vi "ADCS.UnlockECUSecurity.vi"(6 "Diagnostic Protocol":T2, 8 "error in (no error)":errorcluster, 10 "Security":T1={"Source DLL Path"=path "", "Security Level"=1, "Target DLL Path"=path ""}, 11 "diag ref in":T3) -> (0 "error out":errorcluster, 1 "success?":bool, 3 "diag ref out":T3)   [LabVIEW 2015, in "Diagnostics Addon Engine.lvlib"]
uses:
  Diagnostics Addon Engine.lvlib
  <vilib>/Automotive Diagnostic Command Set/Diagnostic Transport.llb/Diag Reference.ctl
  <vilib>/Automotive Diagnostic Command Set/Diagnostic Transport.llb/Transport Protocol Selector.ctl
  <vilib>/Automotive Diagnostic Command Set/Diagnostic Transport.llb/Diag CAN Frame Log.ctl
  Shared/Types/Protocol.ctl
  Shared/Types/Security.ctl
  GMLAN/_SubVIs/SecurityAccess_sendKey.vi
  GMLAN/_SubVIs/SecurityAccess_requestSeed.vi
  <vilib>/Automotive Diagnostic Command Set/Diagnostic Transport.llb/Apply Success Failure Error.vi
  <vilib>/Automotive Diagnostic Command Set/Diagnostic Transport.llb/Diagnostic Service.vi
  GMLAN/GMLAN.lvlib
  <vilib>/addons/Automotive Diagnostic Command Set/NI_Automotive Diagnostic Command Set.lvlib
  Shared/Diagnostics Addon Shared.lvlib
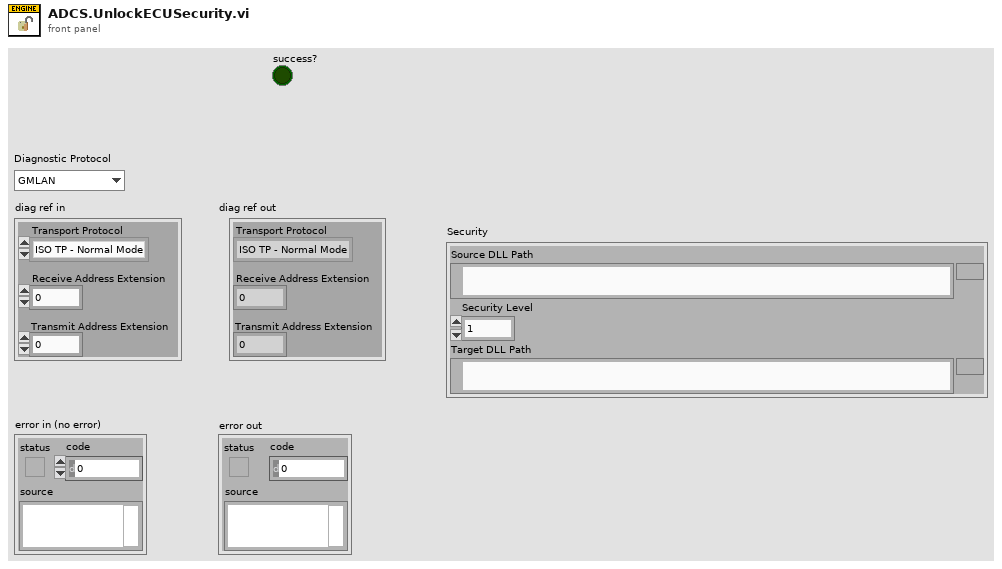
[diagram p1: front panel]
types:
  T1 = typedef "Diagnostics Addon Shared.lvlib/Security.ctl" = cluster{"Source DLL Path":path, "Security Level":u8, "Target DLL Path":path}
  T2 = typedef "Diagnostics Addon Shared.lvlib/Protocol.ctl" = enum16{"GMLAN", "KWP-2000", "UDS", "User-Defined"}
  T3 = typedef "NI_Automotive Diagnostic Command Set.lvlib/Diag Reference.ctl" = cluster{"Diag CAN Handle":u32, "Transport Protocol":T4, "Receive Address Extension":u8, "Transmit Address Extension":u8, "Receive CAN Id":u32, "Transmit CAN Id":u32, "Diag CAN Queue":refnum<queue>, "Log Frames ?":bool, "My TP Address":u8, "Other TP Address":u8, "T1":u16, "T2":u16, "T3":u16, "T4":u16, "Tx SN":u8, "Block Size":u8, "Rx SN":u8, "VW TP Initialized?":bool, "Tx block no":u8, "baud rate":u32, "Interface":string, "Channel Diag CAN Handle":u32, "UDP Connection ID":refnum<k16>, "TCP Connection ID":refnum<k5>, "Target IP Addr":u32, "Source Address":u16, "Target Address":u16, "Send Header NACK?":bool, "DLL Handle":u32, "NAD":u8, "Time Stamp read first":dbl, "Time Stamp read last":dbl, "Time Stamp write first":dbl, "Time Stamp write last":dbl, "Time Stamp write":dbl, "Time Stamp read":dbl}
  T4 = typedef "NI_Automotive Diagnostic Command Set.lvlib/Transport Protocol Selector.ctl" = enum16{"ISO TP - Normal Mode", "ISO TP - Mixed Mode", "VW TP 2.0", "Diagnostics on IP", "ISO TP LIN"}
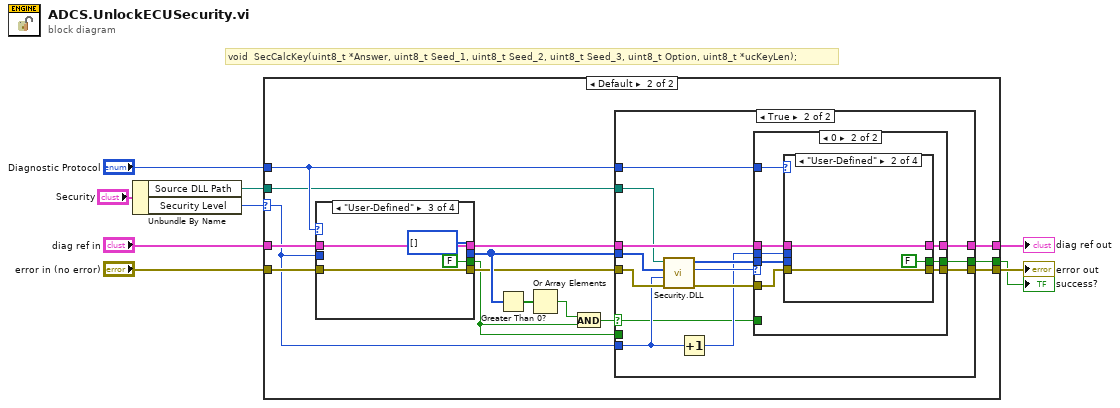
[diagram p0: block diagram]
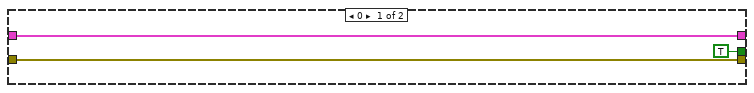
[diagram p2: hidden frame]
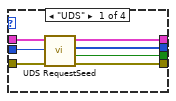
[diagram p3: hidden frame]
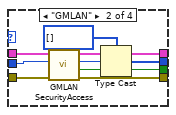
[diagram p4: hidden frame]
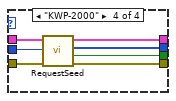
[diagram p5: hidden frame]
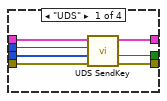
[diagram p8: hidden frame]
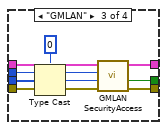
[diagram p9: hidden frame]
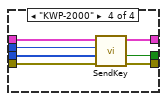
[diagram p10: hidden frame]
diagram:
  # "void  SecCalcKey(uint8_t *Answer, uint8_t Seed_1, uint8_t Seed_2, uint8_t Seed_3, uint8_t Option, uint8_t *ucKeyLen);"
  n1 = Unbundle By Name("Security") -> ("Source DLL Path"=w3:path, "Security Level"=w2:u8)
  n2 = case shown="Default" w2 {
    selector: w2 -> [_ w15]
    tunnel: "diag ref in" -> [w12 w27]
    tunnel: [w12 w26] -> w8
    tunnel: "Diagnostic Protocol" -> [_ w22]
    tunnel: "error in (no error)" -> [w11 w19]
    tunnel: [w11 w17] -> w5
    tunnel: w3 -> [_ w16]
    tunnel: [TRUE ("success?") w13] -> w1
    frame 0 {
    }
    frame Default {
      n3 = case shown="\"User-Defined\"" w22 {
        tunnel: w19 -> [w31 w41 w47 w54]
        tunnel: w27 -> [w32 w43 w46 w53]
        tunnel: [w28 w38 w46 w52] -> w21
        tunnel: w15 -> [w33 w42 _ w51]
        tunnel: [w30 w40 w47 w50] -> w18
        tunnel: [w29 w35 u8[] [] ("seed out") w49] -> w20
        tunnel: [w34 w39 FALSE ("success?") w48] -> w14
        frame "UDS" {
          n4 = call <vilib>:"UDS RequestSeed.vi"("error in (no error)"=w31, "access mode"=w33, "diag ref in"=w32) -> ("error out"=w30:errorcluster, "success?"=w34:bool, "seed out"=w29:u8[], "diag ref out"=w28:T3)  [unwired: 5 in]
        }
        frame "GMLAN" {
          n5 = call-poly "GMLAN SecurityAccess.vi"("error in (no error)"=w41, "subFunction"=w42, "diag ref in"=w43) -> ("error out"=w40:errorcluster, "success?"=w39:bool, "SecuritySeed"=w37:u16, "diag ref out"=w38:T3)  [unwired: 5 in]
          n6 = Type Cast(type=u8[] [] ("seed out"), x=w37) -> (*(type *) &x=w35:u8[])
        }
        frame "User-Defined" {
        }
        frame "KWP-2000" {
          n7 = call <vilib>:"RequestSeed.vi"("error in (no error)"=w54, "access mode"=w51, "diag ref in"=w53) -> ("error out"=w50:errorcluster, "success?"=w48:bool, "seed out"=w49:u8[], "diag ref out"=w52:T3)  [unwired: 5 in]
        }
      }
      n8 = Greater Than 0?(x=w20) -> (x > 0?=w25:bool[])
      n9 = Or Array Elements(Boolean array=w25) -> (logical OR=w23:bool)
      n10 = And(x=w23, y=w14) -> (x .and. y?=w24:bool)
      n11 = case shown="True" w24 {
        selector: w24 -> [_ w59]
        tunnel: [w56 w71] -> w17
        tunnel: w16 -> [_ w65]
        tunnel: w21 -> [w57 w70]
        tunnel: w20 -> [_ w66]
        tunnel: w18 -> [w56 w67]
        tunnel: [w57 w69] -> w26
        tunnel: w15 -> [_ w61]
        tunnel: w22 -> [_ w68]
        tunnel: [w55 w58] -> w13
        tunnel: w14 -> [w55 _]
        frame False {
          # "Positive Response - No Seed\n                   or\nNegative Response"
        }
        frame True {
          n12 = call "Security.DLL.vi"("error in (no error)"=w67, "Option"=w61, "Seed"=w66, "path in"=w65) -> ("error out"=w62:errorcluster, "lockstatus"=w63:u8, "unsigned byte array"=w64:u8[])  [unwired: 5 in]
          n13 = Increment(x=w61) -> (x+1=w60:u8)
          n14 = case shown="0" w63 {
            tunnel: [w74 w82] -> w71
            tunnel: w70 -> [w73 w81]
            tunnel: [w73 w80] -> w69
            tunnel: w60 -> [_ w79]
            tunnel: w68 -> [_ w78]
            tunnel: w62 -> [w74 w77]
            tunnel: w64 -> [_ w76]
            tunnel: [w72 w75] -> w58
            tunnel: w59 -> [w72 _]
            frame Default {
            }
            frame 0 {
              n15 = case shown="\"User-Defined\"" w78 {
                tunnel: [w87 w92 w98 w108] -> w82
                tunnel: w81 -> [w89 w91 w100 w107]
                tunnel: w77 -> [w86 w92 w99 w106]
                tunnel: [w88 w91 w97 w105] -> w80
                tunnel: w79 -> [w84 _ w101 w104]
                tunnel: w76 -> [w85 _ w96 w103]
                tunnel: [w83 FALSE ("success?") w93 w102] -> w75
                frame "UDS" {
                  n16 = call <vilib>:"UDS SendKey.vi"("error in (no error)"=w86, "key in"=w85, "access mode"=w84, "diag ref in"=w89) -> ("error out"=w87:errorcluster, "success?"=w83:bool, "diag ref out"=w88:T3)  [unwired: 5 in]
                }
                frame "User-Defined" {
                }
                frame "GMLAN" {
                  n17 = Type Cast(type=u16 0 ("SecuritySeed"), x=w96) -> (*(type *) &x=w95:u16)
                  n18 = call-poly "GMLAN SecurityAccess.vi"("error in (no error)"=w99, "SecuritySeed"=w95, "subFunction"=w101, "diag ref in"=w100) -> ("error out"=w98:errorcluster, "success?"=w93:bool, "diag ref out"=w97:T3)  [unwired: 5 in]
                }
                frame "KWP-2000" {
                  n19 = call <vilib>:"SendKey.vi"("error in (no error)"=w106, "key in"=w103, "access mode"=w104, "diag ref in"=w107) -> ("error out"=w108:errorcluster, "success?"=w102:bool, "diag ref out"=w105:T3)  [unwired: 5 in]
                }
              }
            }
          }
        }
      }
    }
  }
  "error out" <- w5
  "diag ref out" <- w8
  "success?" <- w1
